vi "data2byte.vi"(8 "argument":dbl, 11 "new function":dbl) -> (0 "protocol":string, 3 "output array":dbl[](array[numeric]))   [LabVIEW 2011]
panel:
  out "msb":dbl
  out "lsb":dbl
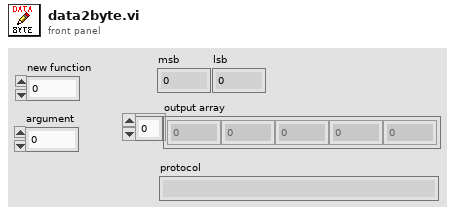
[diagram p1: front panel]
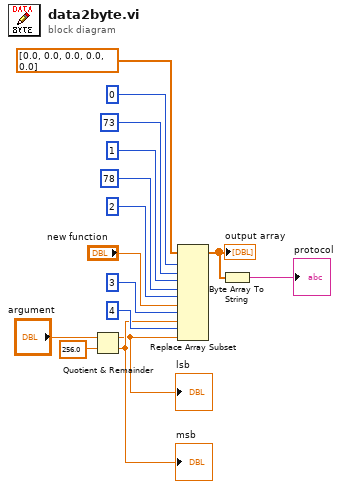
[diagram p0: block diagram]
diagram:
  n1 = Quotient & Remainder(x="argument", y=256.0) -> (x-y*floor(x/y)=w3:dbl, floor(x/y)=w4:dbl)
  "msb" <- w4
  "lsb" <- w3
  n2 = Replace Array Subset(array=dbl[] [0.0, 0.0, 0.0, 0.0, 0.0], new element #1=73 ("function"), index #1=0 ("function"), new element #2=78 ("function"), index #2=1 ("function"), new element #3="new function", index #3=2 ("function"), new element #4=w4, index #4=3 ("MSB"), new element #5=w3, index #5=4 ("LSB")) -> (w2:dbl[])
  "output array" <- w2
  n3 = Byte Array To String(unsigned byte array=w2) -> (string=→"protocol":string)
